vi "setVideoModesAndAtrributes.vi"(8 "error in (no error)":errorcluster, 9 "Attribute Information":T2(array[cluster]), 10 "Video Modes":T3(array[cluster]), 11 "HGF_IMAQDevice in":refnum<class "HGF_IMAQDevice.lvclass">) -> (0 "error out":errorcluster, 3 "HGF_IMAQDevice out":refnum<class "HGF_IMAQDevice.lvclass">)   [LabVIEW 2014, in "HGF_IMAQ.lvlib" / "HGF_IMAQDevice.lvclass"]
doc: "Set available Video Modes and Attribute Informations."
uses:
  HGF_IMAQDevice.lvclass
  <vilib>/vision/driver/IMAQdx.llb/IMAQdx Attribute Type.ctl
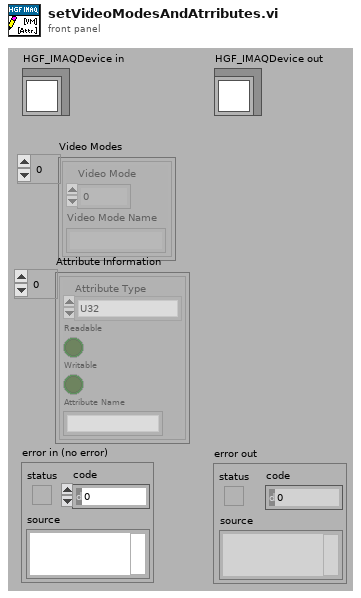
[diagram p1: front panel]
types:
  T1 = typedef "NI_Vision_Acquisition_Software.lvlib/IMAQdx Attribute Type.ctl" = enum32{"U32", "I64", "DBL", "String", "Enum", "Bool", "Command"}
  T2 = cluster{"Attribute Type":T1, "Readable":bool, "Writable":bool, "Attribute Name":string}[]
  T3 = cluster{"Video Mode":u32, "Video Mode Name":string}[]
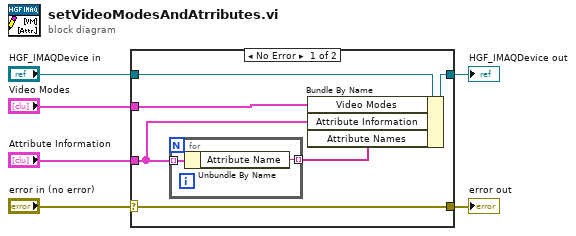
[diagram p0: block diagram]
diagram:
  n1 = case shown="No Error" "error in (no error)" {
    selector: "error in (no error)" -> [w12 w15]
    tunnel: [w12 w15] -> w5
    tunnel: [w10 w16] -> w3
    tunnel: "HGF_IMAQDevice in" -> [w11 w16]
    tunnel: "Video Modes" -> [w9 _]
    tunnel: "Attribute Information" -> [w8 _]
    frame No Error {
      n2 = for {
        tunnel: w8 -> [w14] mode=indexing
        tunnel: [w13] -> w7 mode=indexing
        n3 = Unbundle By Name(w14) -> ("Attribute Name"=w13:string)
      }
      n4 = Bundle By Name(cluster=w11, "Video Modes"=w9, "Attribute Information"=w8, "Attribute Names"=w7) -> (w10:refnum<class "HGF_IMAQDevice.lvclass">)
    }
    frame Error {
    }
  }
  "error out" <- w5
  "HGF_IMAQDevice out" <- w3
